vi "Return VI Path.vi"(10 "name or relative path":string="Data Acq - Simulated.vi") -> (3 "appended path":path)   [LabVIEW 2013]
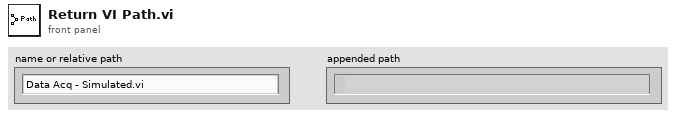
[diagram p1: front panel]
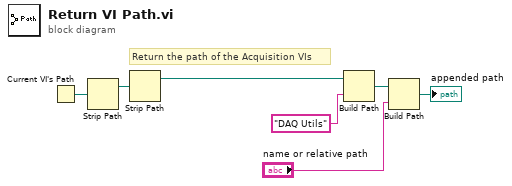
[diagram p0: block diagram]
diagram:
  # "Return the path of the Acquisition VIs"
  n1 = Current VI's Path() -> (path=w7:path)
  n2 = Strip Path(path=w7) -> (stripped path=w2:path)  [unwired: 1 out]
  n3 = Strip Path(path=w2) -> (stripped path=w1:path)  [unwired: 1 out]
  n4 = Build Path(base path=w1, name or relative path="DAQ Utils") -> (appended path=w4:path)
  n5 = Build Path(base path=w4, name or relative path="name or relative path") -> (appended path=→"appended path":path)
